vi "GEOM_MergeLevels.vi"(10 "Array":T1[](array[typedef]) {"fliped" items=["none", "horizontal", "vertical"]; "type" items=["LL", "LR", "UL", "UR"]}) -> (2 "amplifiers 2":T1[][](array[typedef]) {"fliped" items=["none", "horizontal", "vertical"]; "type" items=["LL", "LR", "UL", "UR"]})   [LabVIEW 2016]
uses:
  GEOM_Amplifier.ctl
  GEOM_AmpType.ctl
  GEOM_ROI.ctl
  GEOM_Coords.ctl
panel:
  in  "levels":cluster{"amplifiers":i32, "coord":i32}[](array[cluster])
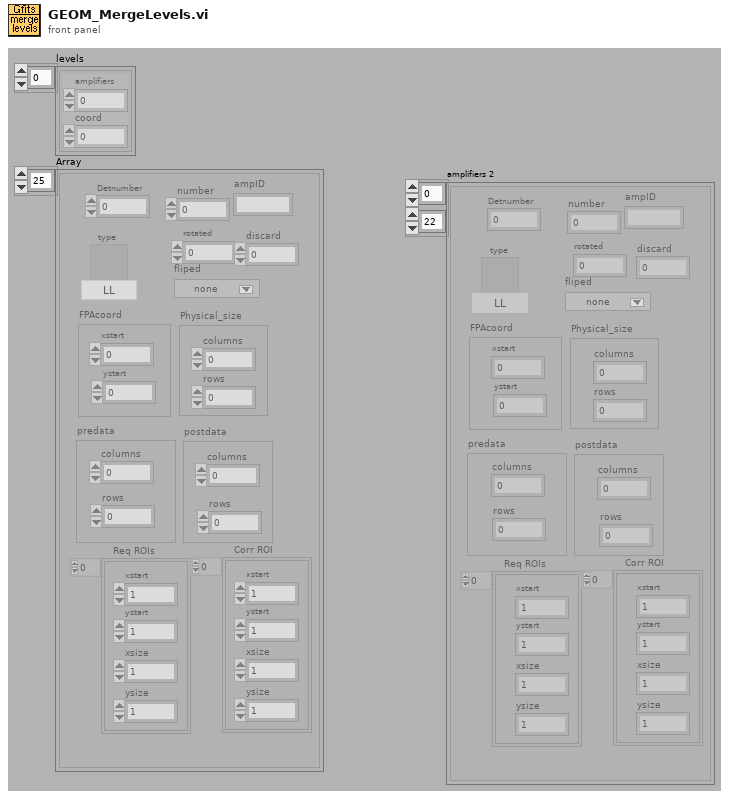
[diagram p1: front panel]
types:
  T1 = typedef "GEOM_Amplifier.ctl" = cluster{"number":i32, "type":T2, "rotated":i16, "fliped":u16, "FPAcoord":cluster{"xstart":i32, "ystart":i32}, "Physical_size":cluster{"columns":i32, "rows":i32}, "predata":cluster{"columns":i32, "rows":i32}, "postdata":cluster{"columns":i32, "rows":i32}, "Req ROIs":T3, "Corr ROI":T3, "Detnumber":i32, "ampID":string, "discard":i32}
  T2 = typedef "GEOM_AmpType.ctl" = u16
  T3 = typedef "GEOM_ROI.ctl" = T4[]
  T4 = typedef "GEOM_Coords.ctl" = cluster{"xstart":u32, "ystart":u32, "xsize":u32, "ysize":u32}
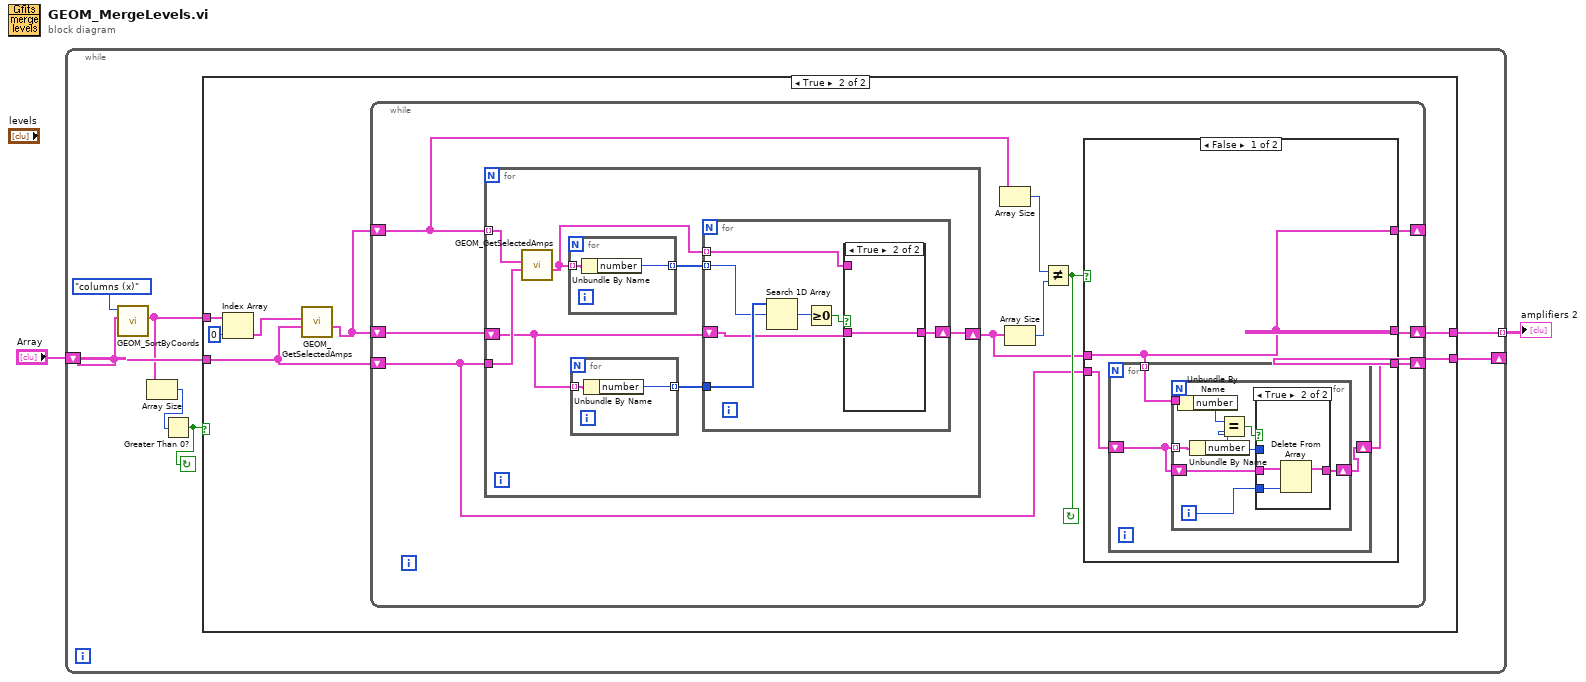
[diagram p0: block diagram]
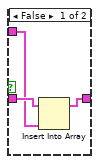
[diagram p3: hidden frame]
diagram:
  n1 = while {
    shift-right: [w7] -> _
    shift-left: "Array" -> [w8]
    tunnel: [w3] -> w1 mode=indexing
    stop <- w4 continue-if-true
    n2 = call "GEOM_SortByCoords.vi"("amplifiers"=w8, "how"=enum16{"rows (y)", "columns (x)"}."columns (x)") -> ("sorted amplifiers"=w6:T1[])  [unwired: 9 out]
    n3 = Array Size(array=w6) -> (size(s)=w5:i32)
    n4 = Greater Than 0?(x=w5) -> (x > 0?=w4:bool)
    n5 = case shown="True" w4 {
      tunnel: w8 -> [w11 w16]
      tunnel: [w11 w14] -> w7
      tunnel: w6 -> [w10 w13]
      tunnel: [w10 w12] -> w3
      frame False {
      }
      frame True {
        n6 = Index Array(array=w13, index=0) -> (element=w17:T1)
        n7 = call "GEOM_GetSelectedAmps.vi"("amplifiers"=w16, "amplifier in"=w17) -> ("selected amplifiers"=w15:T1[])  [unwired: 9 out]
        n8 = while {
          shift-right: [w21] -> w12
          shift-left: w15 -> [w24]
          shift-right: [w19] -> w14
          shift-left: w16 -> [w20]
          shift-right: [w23] -> _
          shift-left: w15 -> [w25]
          stop <- w26 continue-if-true
          n9 = for {
            tunnel: w20 -> [w35]
            tunnel: w25 -> [w34] mode=indexing
            shift-right: [w33] -> w22
            shift-left: w24 -> [w32]
            n10 = call "GEOM_GetSelectedAmps.vi"("amplifiers"=w35, "amplifier in"=w34) -> ("selected amplifiers"=w29:T1[])  [unwired: 9 out]
            n11 = for {
              tunnel: w29 -> [w37] mode=indexing
              tunnel: [w36] -> w30 mode=indexing
              n12 = Unbundle By Name(w37) -> ("number"=w36:i32)
            }
            n13 = for {
              tunnel: w32 -> [w39] mode=indexing
              tunnel: [w38] -> w31 mode=indexing
              n14 = Unbundle By Name(w39) -> ("number"=w38:i32)
            }
            n15 = for {
              shift-right: [w41] -> w33
              shift-left: w32 -> [w42]
              tunnel: w31 -> [w46]
              tunnel: w30 -> [w45] mode=indexing
              tunnel: w29 -> [w40] mode=indexing
              n16 = Search 1D Array(1D array=w46, element=w45) -> (index of element=w44:i32)  [unwired: 1 out]
              n17 = Greater Or Equal To 0?(x=w44) -> (x >= 0?=w43:bool)
              n18 = case shown="True" w43 {
                tunnel: w42 -> [w49 w50]
                tunnel: [w48 w50] -> w41
                tunnel: w40 -> [w47 _]
                frame False {
                  n19 = Insert Into Array(array=w49, new element=w47) -> (w48:T1[])  [unwired: 1 in]
                }
                frame True {
                }
              }
            }
          }
          n20 = Array Size(array=w25) -> (size(s)=w28:i32)
          n21 = Array Size(array=w22) -> (size(s)=w27:i32)
          n22 = Not Equal?(x=w28, y=w27) -> (x != y?=w26:bool)
          n23 = case shown="False" w26 {
            tunnel: [w53 w70] -> w23
            tunnel: w22 -> [w53 w70]
            tunnel: [w53 w70] -> w21
            tunnel: w20 -> [w52 w69]
            tunnel: [w51 w69] -> w19
            frame False {
              n24 = for {
                tunnel: w53 -> [w56] mode=indexing
                shift-right: [w54] -> w51
                shift-left: w52 -> [w55]
                n25 = for {
                  tunnel: w56 -> [w64]
                  tunnel: w55 -> [w63] mode=indexing
                  shift-right: [w59] -> w54
                  shift-left: w55 -> [w60]
                  i -> [w57]
                  n26 = Unbundle By Name(w64) -> ("number"=w61:i32)
                  n27 = Unbundle By Name(w63) -> ("number"=w58:i32)
                  n28 = Equal?(x=w61, y=w58) -> (x = y?=w62:bool)
                  n29 = case shown="True" w62 {
                    tunnel: w60 -> [w65 w68]
                    tunnel: [w65 w66] -> w59
                    tunnel: w58 -> [_ _]
                    tunnel: w57 -> [_ w67]
                    frame False {
                    }
                    frame True {
                      n30 = Delete From Array(array=w68, index=w67) -> (array with subset deleted=w66:T1[])  [unwired: 1 in, 1 out]
                    }
                  }
                }
              }
            }
            frame True {
            }
          }
        }
      }
    }
  }
  "amplifiers 2" <- w1
